vi "DisplayItems.vi"(8 "error in (no error)":errorcluster, 11 "AdvanceTable in":refnum<class "AdvanceTable.lvclass">) -> (0 "error out":errorcluster, 3 "AdvanceTable out":refnum<class "AdvanceTable.lvclass">)   [LabVIEW 2015, in "ActorManagement.lvlib" / "AdvanceTable.lvclass"]
uses:
  AdvanceTable.lvclass
  AdvanceTable.lvclass/AdvanceTable.ctl
  Config/g_tabSetting.vi
  TableItem/TableItem.lvclass
  ActorManagement.lvlib
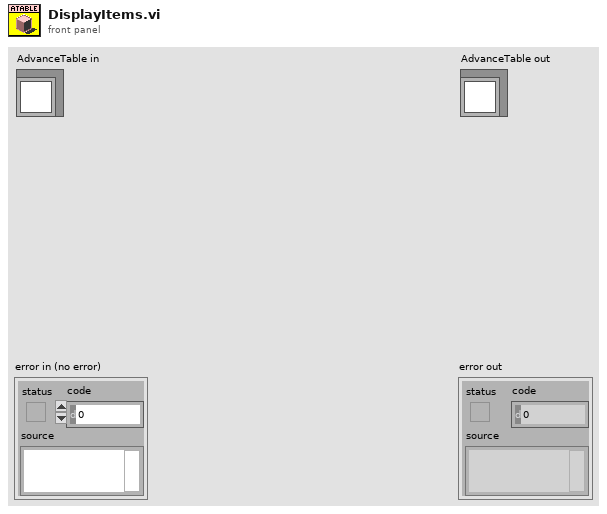
[diagram p1: front panel]
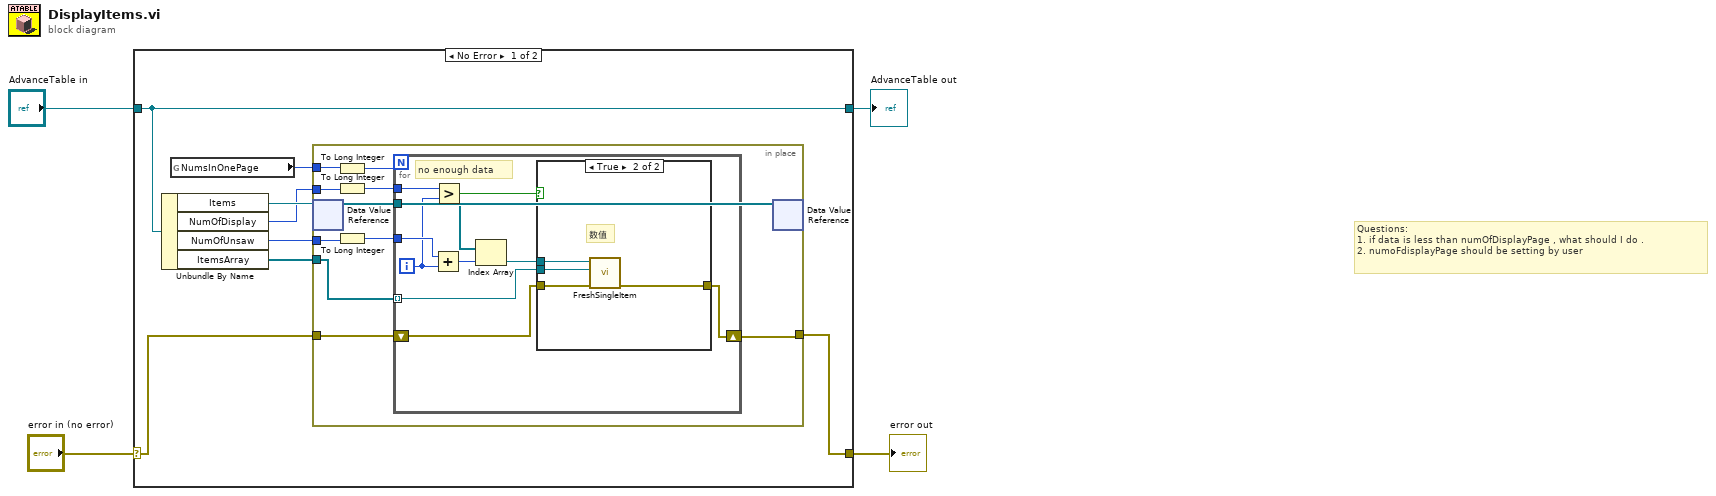
[diagram p0: block diagram]
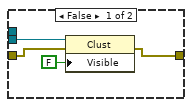
[diagram p2: hidden frame]
diagram:
  # "Questions:\n1. if data is less than numOfDisplayPage , what should I do .\n2. numoFdisplayPage should be setting by user"
  n1 = case shown="No Error" "error in (no error)" {
    selector: "error in (no error)" -> [w7 w42]
    tunnel: [w6 w42] -> w3
    tunnel: [w12 w41] -> w1
    tunnel: "AdvanceTable in" -> [w12 w41]
    frame No Error {
      n2 = Unbundle By Name(w12) -> ("Items"=w11:refnum<data-value>, "NumOfDisplay"=w10:u32, "NumOfUnsaw"=w9:u32, "ItemsArray"=w8:refnum<vi>[])
      n3 = global read "g_tabSetting.vi" "NumsInOnePage"() -> (w5:u32)
      n4 = in-place {
        in-place-border: w10 -> [w16]
        in-place-border: w9 -> [w18]
        in-place-border: w8 -> [w22]
        in-place-border: w7 -> [w21]
        in-place-border: [w19] -> w6
        in-place-border: w5 -> [w14]
        n5 = in-place-dvr #1(w11) -> (w20:refnum<class "TableItem.lvclass">[])  [unwired: 1 out]
        n6 = To Long Integer(number=w14) -> (32bit integer=w13:i32)
        n7 = To Long Integer(number=w16) -> (32bit integer=w15:i32)
        n8 = To Long Integer(number=w18) -> (32bit integer=w17:i32)
        n9 = for {
          N: w13 -> [_]
          tunnel: w20 -> [w32]
          tunnel: w22 -> [w29] mode=indexing
          shift-right: [w26] -> w19
          shift-left: w21 -> [w28]
          tunnel: w17 -> [w27]
          tunnel: w15 -> [w25]
          i -> [w24]
          # "no enough data"
          n10 = Add(x=w27, y=w24) -> (x+y=w31:i32)
          n11 = Greater?(x=w25, y=w24) -> (0:w23:bool)
          n12 = Index Array(array=w32, index=w31) -> (element=w30:refnum<class "TableItem.lvclass">)
          n13 = case shown="True" w23 {
            tunnel: w30 -> [_ w40]
            tunnel: w29 -> [w36 w39]
            tunnel: w28 -> [w35 w38]
            tunnel: [w33 w37] -> w26
            frame False {
              n14 = property class="Clust"(reference=w36, error in=w35, "Visible"=FALSE) -> (error out=w33:errorcluster)  [unwired: 1 out]
            }
            frame True {
              # "数值"
              n15 = call-dynamic "FreshSingleItem.vi"("error in (no error)"=w38, "TableItem"=w39, "TableItem in"=w40) -> ("error out"=w37:errorcluster)  [unwired: 7 in, 1 out]
            }
          }
        }
        n16 = in-place-dvr #1(w20) -> ()  [unwired: 2 out]
      }
    }
    frame Error {
    }
  }
  "error out" <- w3
  "AdvanceTable out" <- w1
